vi "dfd_Dummy_INT Filtering wStateA.vi"(9 "state in":i32[](array[numeric]), 11 "x":i16) -> (1 "state out":i32[](array[numeric]), 3 "y":i16)   [LabVIEW 2017]
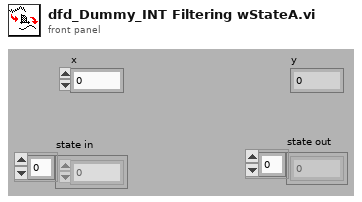
[diagram p1: front panel]
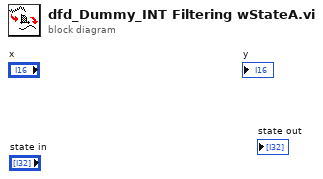
[diagram p0: block diagram]
diagram:
